vi "final.vi"() -> ()   [LabVIEW 2013]
panel:
  out "INDICATOR":T1
  out "BUFFER":T2
  out "DX":T2
  out "CX":T2
  out "BX":T2
  out "AX":T2
  out "OVERFLOW":bool
  in  "KEYBOARD":T3
  in  "reset registers":bool
  in  "tick":bool
  in  "FROM":cluster{"c2":bool, "c1":bool, "c0":bool}
  in  "TO":cluster{"c2":bool, "c1":bool, "c0":bool}
  in  "OPERATION":T4
  out "OUT":T2
  out "INPUT":T5
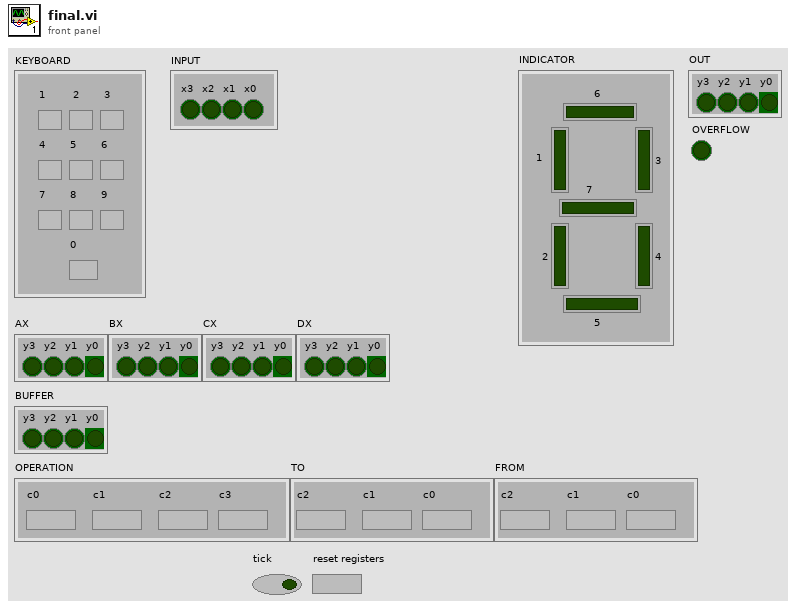
[diagram p1: front panel]
types:
  T1 = cluster{"6":bool, "3":bool, "1":bool, "7":bool, "2":bool, "4":bool, "5":bool}
  T2 = cluster{"y3":bool, "y2":bool, "y1":bool, "y0":bool}
  T3 = cluster{"1":bool, " 2":bool, " 3":bool, "4":bool, "5":bool, "6":bool, "7":bool, "8":bool, "9":bool, "0":bool}
  T4 = cluster{"c0":bool, "c1":bool, "c2":bool, "c3":bool}
  T5 = cluster{"x3":bool, "x2":bool, "x1":bool, "x0":bool}
  T6 = cluster{"y0":bool, "y1":bool, "y2":bool, "y3":bool}
  T7 = cluster{"AX":cluster{"y3":bool, "y2":bool, "y1":bool, "y0":bool}, "BX":cluster{"y3":bool, "y2":bool, "y1":bool, "y0":bool}, "CX":cluster{"y3":bool, "y2":bool, "y1":bool, "y0":bool}, "DX":cluster{"y3":bool, "y2":bool, "y1":bool, "y0":bool}, "OUT":cluster{"y3":bool, "y2":bool, "y1":bool, "y0":bool}}
  T8 = cluster{"ax":bool, "bx":bool, "cx":bool, "dx":bool}
  T9 = cluster{"OUTPUT":cluster{"y3":bool, "y2":bool, "y1":bool, "y0":bool}, "OUTPUT":cluster{"y3":bool, "y2":bool, "y1":bool, "y0":bool}, "OUTPUT":cluster{"y3":bool, "y2":bool, "y1":bool, "y0":bool}, "OUTPUT":cluster{"y3":bool, "y2":bool, "y1":bool, "y0":bool}}
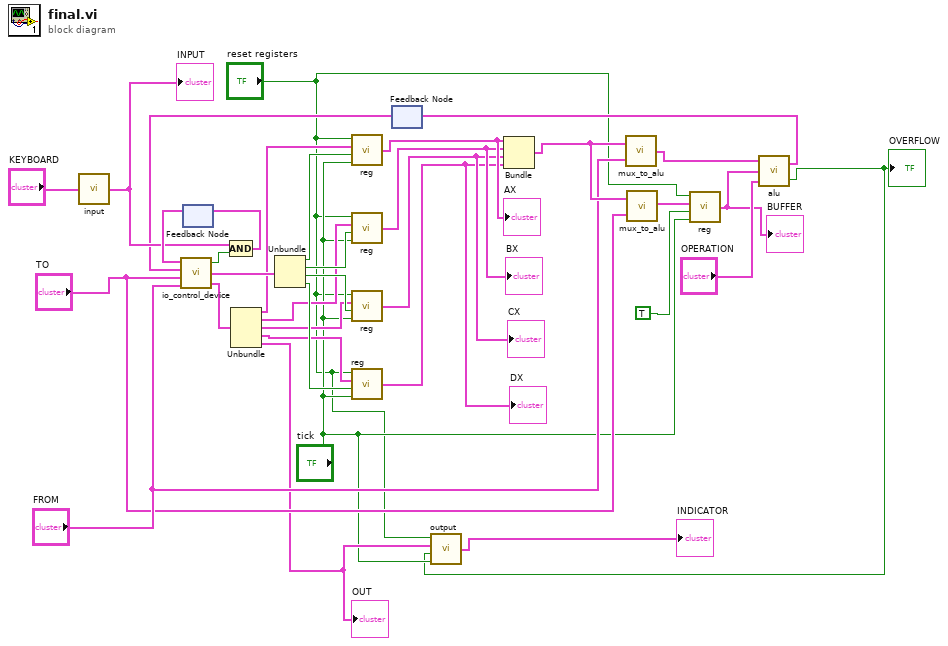
[diagram p0: block diagram]
diagram:
  n1 = call "input.vi"("INPUT"="KEYBOARD") -> ("OUTPUT"=w21:T6)
  "INPUT" <- w21
  n2 = feedback #1() -> (w27:T6)  [unwired: 1 in]
  n3 = feedback #2() -> (w7:T2)  [unwired: 1 in]
  n4 = call "io_control_device.vi"("FROM"="FROM", "TO"="TO", "INPUT_REGS"=w7, "INPUT_KEYBOARD"=w27) -> ("OUTPUT"=w26:T7, "WRITE"=w30:T8, "KEYBOARD_IS_ON"=w29:bool)
  n5 = Compound Arithmetic op=AND(w21, w29) -> (w28:T6)
  n6 = feedback-in #1(w28) -> ()
  n7 = Unbundle(w26) -> ("AX"=w20:T2, "BX"=w25:T2, "CX"=w24:T2, "DX"=w23:T2, "OUT"=w5:T2)
  "OUT" <- w5
  n8 = Unbundle(w30) -> ("ax"=w34:bool, "bx"=w33:bool, "cx"=w32:bool, "dx"=w31:bool)
  n9 = call "reg.vi"("C"="tick", "WRITE"=w34, "INPUT"=w20, "R"="reset registers") -> ("OUTPUT"=w19:T2)
  "AX" <- w19
  n10 = call "reg.vi"("C"="tick", "WRITE"=w33, "INPUT"=w25, "R"="reset registers") -> ("OUTPUT"=w18:T2)
  "BX" <- w18
  n11 = call "reg.vi"("C"="tick", "WRITE"=w32, "INPUT"=w24, "R"="reset registers") -> ("OUTPUT"=w17:T2)
  "CX" <- w17
  n12 = call "reg.vi"("C"="tick", "WRITE"=w31, "INPUT"=w23, "R"="reset registers") -> ("OUTPUT"=w16:T2)
  "DX" <- w16
  n13 = Bundle("OUTPUT"=w19, "OUTPUT"=w18, "OUTPUT"=w17, "OUTPUT"=w16) -> (w12:T9)  [unwired: 1 in]
  n14 = call "mux_to_alu.vi"("CONTROL"="FROM", "INPUT"=w12) -> ("OUTPUT"=w15:T2)
  n15 = call "mux_to_alu.vi"("CONTROL"="TO", "INPUT"=w12) -> ("OUTPUT"=w13:T2)
  n16 = call "reg.vi"("C"="tick", "WRITE"=TRUE, "INPUT"=w13, "R"="reset registers") -> ("OUTPUT"=w9:T2)
  "BUFFER" <- w9
  n17 = call "alu.vi"("CONTROL"="OPERATION", "INPUT_B"=w9, "INPUT_A"=w15) -> ("OVERFLOW"=w2:bool, "OUTPUT"=w8:T2)
  "OVERFLOW" <- w2
  n18 = feedback-in #2(w8) -> ()
  n19 = call "output.vi"("C"="tick", "OVERFLOW"=w2, "INPUT"=w5, "R"="reset registers") -> ("OUTPUT"=→"INDICATOR":T1)
